vi "IP Adress Init.vi"(3 "Container State":T3 caption="容器状态", 4 "Previous State":variant caption="前期状态", 5 "Previous Version":T2 caption="前期版本") -> (2 "Current State":T1={"Front Color"=1985280, "User Event"=refnum} caption="当前状态")   [LabVIEW 2013, in "IP Adresss Control.xctl"]
uses:
  IP Adresss Control.xctl
  IP Address Status.ctl
  UserEvent/IP User Event.ctl
  <vilib>/_xctls/Container State.ctl
  <vilib>/_xctls/Version.ctl
  <vilib>/_xctls/XControlSupport.lvlib
panel:
  in  "Default Indicator State":T1={"Front Color"=1985280, "User Event"=refnum} caption="默认显示控件状态"
  in  "Default Control State":T1={"Front Color"=1985280, "User Event"=refnum} caption="默认输入控件状态"
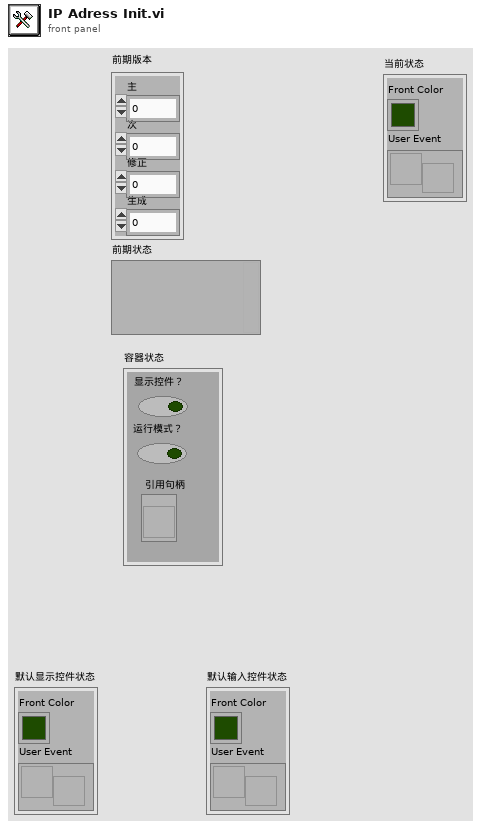
[diagram p1: front panel]
types:
  T1 = typedef "IP Adresss Control.xctl/IP Address Status.ctl" = cluster{"Front Color":u32, "User Event":refnum<user-event>}
  T2 = typedef "XControlSupport.lvlib/Version.ctl" = cluster{"Major":u16, "Minor":u16, "Fix":u16, "Build":u16}
  T3 = typedef "XControlSupport.lvlib/Container State.ctl" = cluster{"Indicator?":bool, "Run Mode?":bool, " Refnum":refnum<vi>}
  T4 = typedef "IP Adresss Control.xctl/IP User Event.ctl" = cluster{"Message":string}
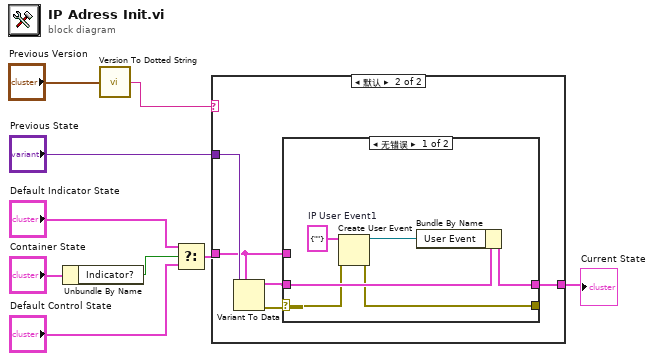
[diagram p0: block diagram]
diagram:
  n1 = Unbundle By Name("Container State") -> ("Indicator?"=w4:bool)
  n2 = call <vilib>:"Version To Dotted String.vi"("Version"="Previous Version") -> ("String Version"=w1:string)
  n3 = Select(t="Default Indicator State", s=w4, f="Default Control State") -> (s? t:f=w3:T1)
  n4 = case shown="默认" w1 {
    tunnel: "Previous State" -> [_ w15]
    tunnel: [w10 w11] -> w8
    tunnel: w3 -> [w10 w12]
    frame "0.0.0.0" {
      # "已创建，并使用默认状态"
    }
    frame Default {
      n5 = Variant To Data(type=w12, Variant=w15) -> (data=w13:T1, error out=w14:errorcluster)  [unwired: 1 in]
      n6 = case shown="无错误" w14 {
        selector: w14 -> [w19 w22]
        tunnel: w13 -> [w21 _]
        tunnel: [w17 w23] -> w11
        tunnel: w12 -> [_ w23]
        tunnel: [w18 w22] -> _
        frame No Error {
          w20 = T4 {"Message"=""}  # IP User Event1
          n7 = Create User Event(user event datatype=w20, error in=w19) -> (user event=w16:refnum<user-event>, error out=w18:errorcluster)
          n8 = Bundle By Name(cluster=w21, "User Event"=w16) -> (w17:T1)
        }
        frame Error {
          # "转换前期保存状态时\n发生错误。使用默认。"
        }
      }
    }
  }
  "Current State" <- w8
